vi "Fetch.vi"   [LabVIEW 2012, in "NH Research Regenerative Test Series.lvlib"]
doc: "This returns previously acquired data for single measurements via Fetch commands."
uses:
  <instrlib>/NH Research Regenerative Test Series/NH Research Regenerative Test Series.lvlib
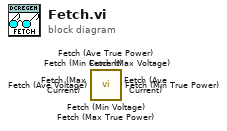
[diagram p0: block diagram]
diagram:
  n1 = call <instrlib>:"Fetch (Min Voltage).vi"() -> ()  [unwired: 13 in, 3 out]
  n2 = call <instrlib>:"Fetch (Max Voltage).vi"() -> ()  [unwired: 13 in, 3 out]
  n3 = call <instrlib>:"Fetch (Ave Voltage).vi"() -> ()  [unwired: 13 in, 3 out]
  n4 = call <instrlib>:"Fetch (Min True Power).vi"() -> ()  [unwired: 13 in, 3 out]
  n5 = call <instrlib>:"Fetch (Max True Power).vi"() -> ()  [unwired: 13 in, 3 out]
  n6 = call <instrlib>:"Fetch (Ave True Power).vi"() -> ()  [unwired: 13 in, 3 out]
  n7 = call <instrlib>:"Fetch (Min Current).vi"() -> ()  [unwired: 13 in, 3 out]
  n8 = call <instrlib>:"Fetch (Max Current).vi"() -> ()  [unwired: 13 in, 3 out]
  n9 = call <instrlib>:"Fetch (Ave Current).vi"() -> ()  [unwired: 13 in, 3 out]
